vi "Truncate CAN DLC.vi"(10 "DLC in":u32, 11 "IO Mode":enum32{"CAN", "CAN FD", "CAN FD + BRS"}(ring)) -> (3 "DLC out":u32)   [LabVIEW 2025, in "CAN-LIN Frame Generator.lvclass"]
uses:
  CAN-LIN Frame Generator.lvclass
  CAN-LIN Frame Generator.lvclass/CAN-LIN Frame Generator.ctl
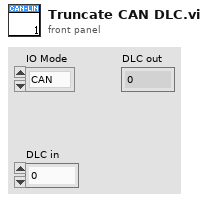
[diagram p1: front panel]
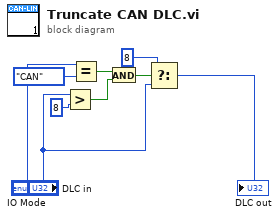
[diagram p0: block diagram]
diagram:
  n1 = Greater?(x="DLC in", y=u32 8) -> (0:w5:bool)
  n2 = Equal?(x="IO Mode", y=enum32{"CAN", "CAN FD", "CAN FD + BRS"}."CAN") -> (x = y?=w3:bool)
  n3 = And(x=w3, y=w5) -> (x .and. y?=w6:bool)
  n4 = Select(t=u32 8, s=w6, f="DLC in") -> (s? t:f=→"DLC out":u32)
